vi "Perform Fast Buffer Task.vi"(8 "error in (no error)":errorcluster, 11 "Calling Actor in":refnum<class "Calling Actor.lvclass">) -> (0 "error out":errorcluster, 3 "Calling Actor out":refnum<class "Calling Actor.lvclass">)   [LabVIEW 2020, in "Calling Actor.lvlib" / "Calling Actor.lvclass"]
uses:
  Calling Actor.lvclass
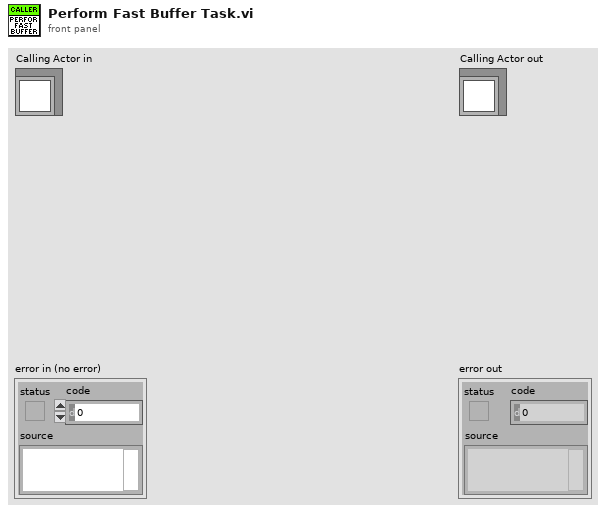
[diagram p1: front panel]
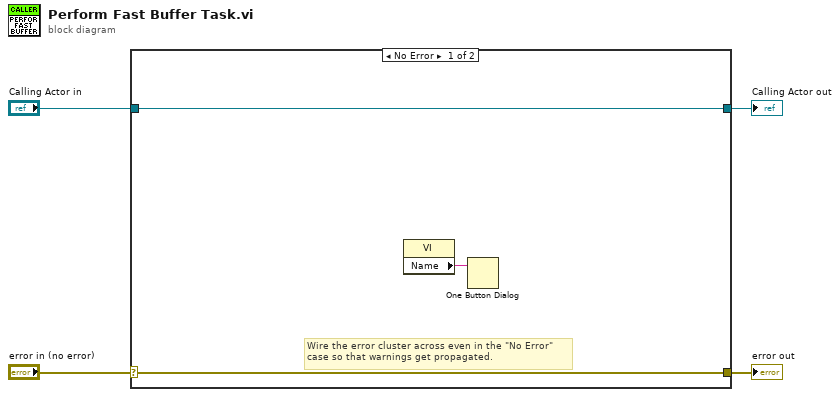
[diagram p0: block diagram]
diagram:
  n1 = case shown="No Error" "error in (no error)" {
    selector: "error in (no error)" -> [w6 w9]
    tunnel: [w6 w9] -> w3
    tunnel: [w7 w8] -> w1
    tunnel: "Calling Actor in" -> [w7 w8]
    frame No Error {
      # "Wire the error cluster across even in the \"No Error\"\ncase so that warnings get propagated."
      n2 = property class="VI"() -> ("Name"=w5:string)  [unwired: 2 in, 2 out]
      n3 = One Button Dialog(message=w5) -> ()  [unwired: 1 in, 1 out]
    }
    frame Error {
    }
  }
  "error out" <- w3
  "Calling Actor out" <- w1
